vi "ExecuteMethod.vi"(6 "AsyncError":refnum<queue>, 7 "LabVIEWObjectIn":refnum<class>, 10 "VIIn":refnum<vi>, 11 "QueueDataIn":T1) -> (0 "ReplyData":variant, 1 "AsyncErrorOut":errorcluster, 2 "MethodErrorOut":errorcluster, 3 "VICallErrorOut":errorcluster, 4 "Exit":bool, 5 "LabVIEWObjectOut":refnum<class>)   [LabVIEW 2021, in "YActor.lvclass"]
uses:
  YActor.lvclass
  CmdCtrl.ctl
  AsyncErrorHandling.ctl
  CallMode.ctl
  RawTrace.vi
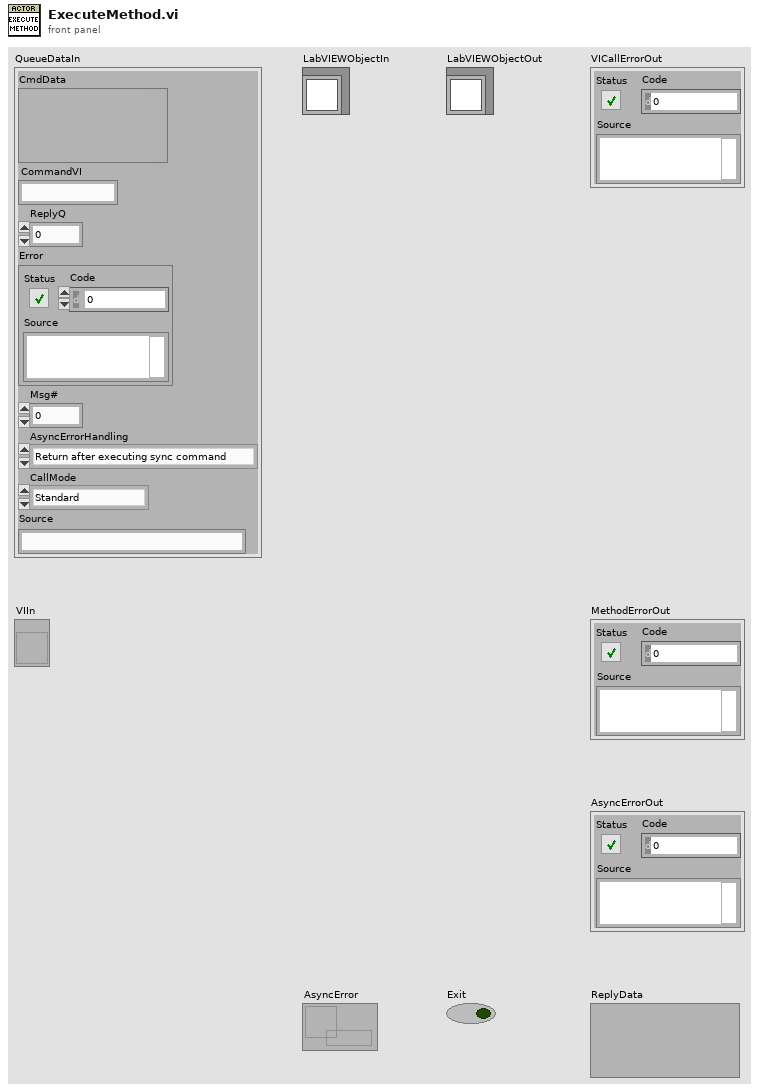
[diagram p1: front panel]
types:
  T1 = typedef "YActor.lvclass/CmdCtrl.ctl" = cluster{"CmdData":variant, "CommandVI":string, "ReplyQ":i64, "Error":errorcluster, "Msg#":u32, "AsyncErrorHandling":T2, "CallMode":T3, "Source":string}
  T2 = typedef "YActor.lvclass/AsyncErrorHandling.ctl" = enum16{"Return after executing sync command", "Return before executing sync command", "Don't return error"}
  T3 = typedef "YActor.lvclass/CallMode.ctl" = enum16{"Standard", "Call&Collect"}
  T4 = cluster{"seconds since 1Jan1904":timestamp, "seconds since 1Jan1904":timestamp}
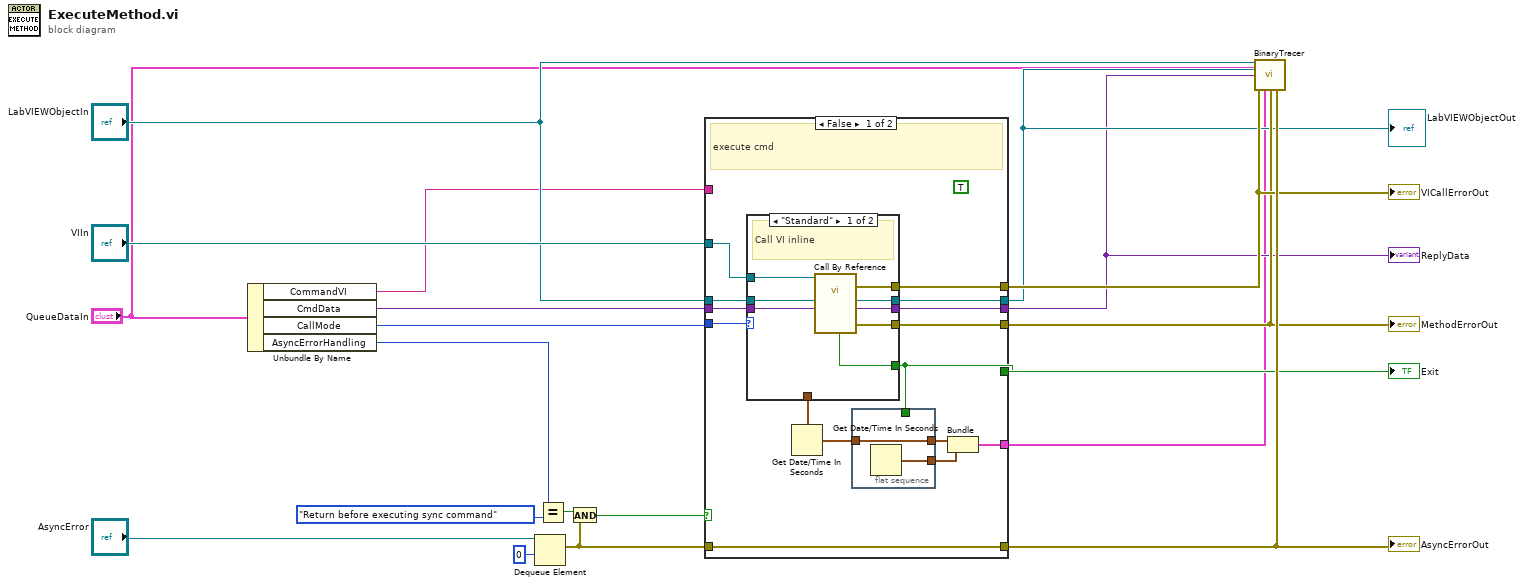
[diagram p0: block diagram]
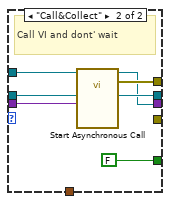
[diagram p2: hidden frame]
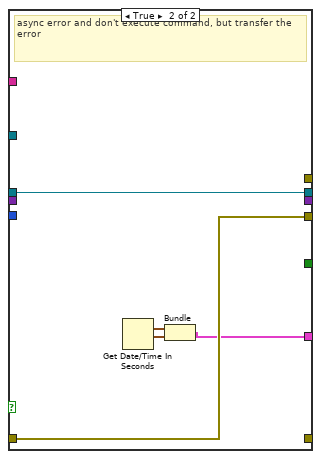
[diagram p3: hidden frame]
diagram:
  n1 = Unbundle By Name("QueueDataIn") -> ("CommandVI"=w1:string, "CmdData"=w9:variant, "CallMode"=w8:T3, "AsyncErrorHandling"=w7:T2)
  n2 = Dequeue Element(queue="AsyncError", timeout in ms (-1)=0) -> (element=w20:errorcluster)  [unwired: 1 in, 3 out]
  n3 = Equal?(x=w7, y=AsyncErrorHandling."Return before executing sync command" ("x")) -> (x = y?=w13:bool)
  n4 = And(x=w13, y=w20) -> (x .and. y?=w14:bool)
  n5 = case shown="False" w14 {
    tunnel: [w31 _] -> w3
    tunnel: [w32 w54] -> w17
    tunnel: "VIIn" -> [w30 _]
    tunnel: w9 -> [w29 _]
    tunnel: [w25 _] -> w11
    tunnel: [w34 _] -> w18
    tunnel: [w28 w53] -> w5
    tunnel: "LabVIEWObjectIn" -> [w27 w53]
    tunnel: w8 -> [w26 _]
    tunnel: w20 -> [w33 w54]
    tunnel: [w33 _] -> w19
    tunnel: [w21 w51] -> w2
    tunnel: w1 -> [_ _]
    frame False {
      (unwired) TRUE ("MergeErrors")
      # "execute cmd"
      n6 = Get Date/Time In Seconds() -> (seconds since 1Jan1904=w24:timestamp)
      n7 = case shown="\"Standard\"" w26 {
        tunnel: [w42 w45] -> w31
        tunnel: [w44 _] -> w32
        tunnel: w30 -> [w41 w49]
        tunnel: w29 -> [w40 w48]
        tunnel: [w39 FALSE ("Exit")] -> w25
        tunnel: [w43 w50] -> w34
        tunnel: [w38 w47] -> w28
        tunnel: w27 -> [w37 w47]
        tunnel: w24 -> [_ _]
        frame "Standard" {
          # "Call VI inline"
          n8 = call-by-ref "?"(reference=w41, "Cmd Data"=w40, "Local in"=w37) -> (error out=w43:errorcluster, 0:"error out"=w44:errorcluster, "Reply Data"=w42:variant, "Local out"=w38:refnum<class>, "Exit"=w39:bool)  [unwired: 7 in, 1 out]
        }
        frame "Call&Collect" {
          # "Call VI and dont' wait"
          n9 = call-by-ref "Start Asynchronous Call"(reference=w49, "Cmd Data"=w48, "Local in"=w47) -> (reference out=w45:refnum<vi>, error out=w50:errorcluster)  [unwired: 7 in, 4 out]
        }
      }
      n10 = flat-sequence {
        tunnel: w25 -> [_]
        tunnel: [w36] -> w23
        tunnel: w24 -> [w36]
        tunnel: [w35] -> w22
        frame #0 {
          n11 = Get Date/Time In Seconds() -> (seconds since 1Jan1904=w35:timestamp)
        }
      }
      n12 = Bundle("seconds since 1Jan1904"=w23, "seconds since 1Jan1904"=w22) -> (w21:T4)  [unwired: 1 in]
    }
    frame True {
      # "async error and don't execute command, but transfer the error"
      n13 = Get Date/Time In Seconds() -> (seconds since 1Jan1904=w52:timestamp)
      n14 = Bundle("seconds since 1Jan1904"=w52, "seconds since 1Jan1904"=w52) -> (w51:T4)  [unwired: 1 in]
    }
  }
  "ReplyData" <- w3
  "LabVIEWObjectOut" <- w5
  "Exit" <- w11
  "MethodErrorOut" <- w17
  "AsyncErrorOut" <- w19
  "VICallErrorOut" <- w18
  n15 = call "BinaryTracer.vi"("YActorIn"="LabVIEWObjectIn", "QueueData"="QueueDataIn", "MethodDataOutput"=w5, "ReplyData"=w3, "MethodErrorIn"=w18, "Timing"=w2, "MethodCallError"=w17, "AsyncError"=w19) -> ()  [unwired: 7 in, 1 out]
